vi "Do Request.vi"(7 "Processing In":refnum<class "Processing.lvclass">, 11 "Test Sessions Controller in":refnum<class "Test Sessions Controller.lvclass">) -> (0 "error out":errorcluster, 5 "Processing":refnum<class "Processing.lvclass">)   [LabVIEW 2020, in "Test Sessions Controller.lvclass"]
uses:
  Test Sessions Controller.lvclass
  Test Sessions Controller.lvclass/Test Sessions Controller.ctl
  lv-http-server/HTTP Server/Session/Session.lvclass
  lv-http-util/HTTP Utils/Request/Request.lvclass
  lv-stream/stream/URI/URI.lvclass
  lv-http-util/HTTP Utils/Response/Response.lvclass
  lv-http-server/HTTP Server/Processing/Processing.lvclass
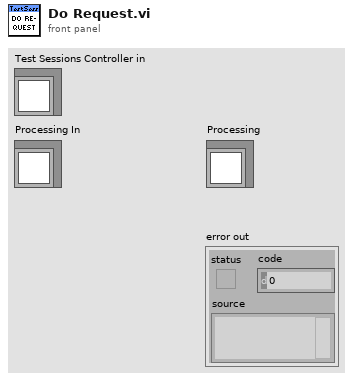
[diagram p1: front panel]
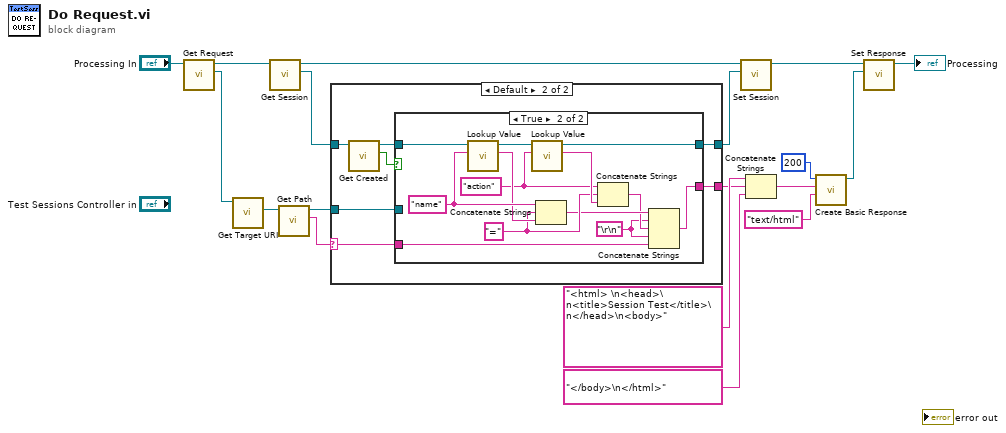
[diagram p0: block diagram]
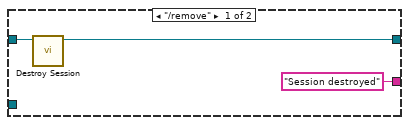
[diagram p2: hidden frame]
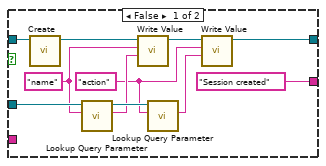
[diagram p3: hidden frame]
diagram:
  n1 = call "Get Request.vi"("Processing in"="Processing In") -> ("Request"=w6:refnum<class "Request.lvclass">, "Processing out"=w5:refnum<class "Processing.lvclass">)  [unwired: 9 in]
  n2 = call "Get Target URI.vi"("Request in"=w6) -> ("Target URI"=w18:refnum<class "URI.lvclass">)  [unwired: 8 in, 2 out]
  n3 = call "Get Session.vi"("Processing in"=w5) -> ("Session"=w9:refnum<class "Session.lvclass">, "Processing out"=w7:refnum<class "Processing.lvclass">)  [unwired: 9 in]
  n4 = call "Get Path.vi"("URI in"=w18) -> ("Path"=w16:string, "URI out"=w17:refnum<class "URI.lvclass">)  [unwired: 8 in, 1 out]
  n5 = case shown="Default" w16 {
    selector: w16 -> [_ w22]
    tunnel: w9 -> [w20 w28]
    tunnel: w17 -> [_ w25]
    tunnel: [w19 w24] -> w8
    tunnel: ["Session destroyed" ("Name") w23] -> w10
    frame "/remove" {
      n6 = call "Destroy Session.vi"("Session in"=w20) -> ("Session out"=w19:refnum<class "Session.lvclass">)  [unwired: 9 in, 1 out]
    }
    frame Default {
      n7 = call "Get Created.vi"("Session in"=w28) -> ("Created"=w27:bool, "Session out"=w26:refnum<class "Session.lvclass">)  [unwired: 8 in, 1 out]
      n8 = case shown="True" w27 {
        tunnel: w26 -> [w37 w52]
        tunnel: w25 -> [w39 _]
        tunnel: [w30 w50] -> w24
        tunnel: ["Session created" ("Name") w42] -> w23
        tunnel: w22 -> [_ w40]
        frame False {
          w31 = "action" ("Name")
          w35 = "name" ("Name")
          n9 = call "Create.vi"("Session in"=w37) -> ("Session out"=w36:refnum<class "Session.lvclass">)  [unwired: 9 in, 1 out]
          n10 = call "Lookup Query Parameter.vi"("Name"=w35, "URI in"=w39) -> ("Value"=w34:string, "URI out"=w38:refnum<class "URI.lvclass">)  [unwired: 6 in, 2 out]
          n11 = call "Write Value.vi"("Value"=w34, "Name"=w35, "Session in"=w36) -> ("Session out"=w33:refnum<class "Session.lvclass">)  [unwired: 6 in, 2 out]
          n12 = call "Lookup Query Parameter.vi"("Name"=w31, "URI in"=w38) -> ("Value"=w32:string)  [unwired: 6 in, 3 out]
          n13 = call "Write Value.vi"("Value"=w32, "Name"=w31, "Session in"=w33) -> ("Session out"=w30:refnum<class "Session.lvclass">)  [unwired: 6 in, 2 out]
        }
        frame True {
          w41 = "\r\n"
          w45 = "=" ("string")
          w46 = "action" ("Name")
          w49 = "name" ("Name")
          n14 = call "Lookup Value.vi"("Name"=w49, "Session in"=w52) -> ("Value"=w48:string, "Session out"=w51:refnum<class "Session.lvclass">)  [unwired: 6 in, 2 out]
          n15 = call "Lookup Value.vi"("Name"=w46, "Session in"=w51) -> ("Value"=w47:string, "Session out"=w50:refnum<class "Session.lvclass">)  [unwired: 6 in, 2 out]
          n16 = Concatenate Strings(w49, w45, w48) -> (w44:string)
          n17 = Concatenate Strings(w46, w45, w47) -> (w43:string)
          n18 = Concatenate Strings(w44, w41, w43, w41, w40) -> (w42:string)
        }
      }
    }
  }
  n19 = call "Set Session.vi"("Session"=w8, "Processing in"=w7) -> ("Processing out"=w3:refnum<class "Processing.lvclass">)  [unwired: 9 in]
  n20 = Concatenate Strings("<html> \n<head>\n<title>Session Test</title>\n</head>\n<body>", w10, "</body>\n</html>") -> (w11:string)
  n21 = call "Create Basic Response.vi"("Content-Type (text/plain)"="text/html", "Payload"=w11, "Status Code"=u16 200) -> ("Response out"=w2:refnum<class "Response.lvclass">)  [unwired: 7 in, 1 out]
  n22 = call "Set Response.vi"("Response"=w2, "Processing in"=w3) -> ("Processing out"=→"Processing":refnum<class "Processing.lvclass">)  [unwired: 9 in]
